vi "RSNRPZ Get Usage Map.vi"(8 "error in (no error)":errorcluster, 9 "Max Len (1024)":u32=1024) -> (0 "error out":errorcluster, 1 "Map":string, 2 "Ret Len":u32)   [LabVIEW 2010]
doc: "Starting with revision 3.2.1.0 of this driver, the underlying low level library has been made usable by multiple applications concurrently. A sensor which is already in use by another running application cannot by initialized by a different In this case the rsnrpz_init() function would return a status NRP_ERROR_SENSOR_IN_USE (0xC0000022). \n\nrsnrpz_getUsageMap() can be used to get a textual description of the current sensor & application relationship. For a sensor which is already in use, the application which holds the sensor, is shown in the usage map. This information can, for example, be presented to a user. \n\nThe textual usage map is returned via a char buffer 'Map' which should be supplied by the caller. 'maxLen' should be set to the size of the user's buffer in order to limit the amount of data which will be copied to 'map'.\nIf 'Ret Len' is not NULL, the current length of the usage map is returned here (which may be longer than 'Max Len'."
uses:
  rsnrpz_32.dll
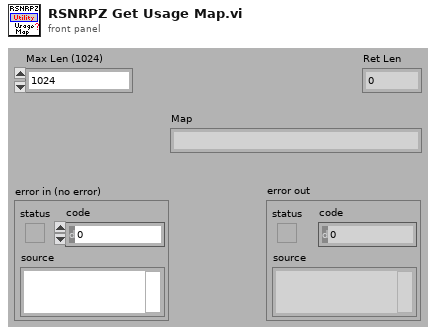
[diagram p1: front panel]
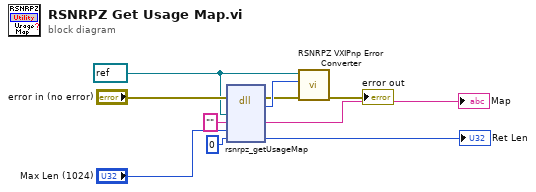
[diagram p0: block diagram]
diagram:
  w1 = refnum<visa-resource-name> refnum ("dup VISA session")
  n1 = dll-call lib="rsnrpz_32.dll" fn="rsnrpz_getUsageMap"(error in="error in (no error)", "Instrument Handle"=w1, "Map"="", "Max Len"="Max Len (1024)", "Ret Len"=u32 0) -> (error out=w4:errorcluster, w7:i32, "Map"=→"Map":string, "Ret Len"=→"Ret Len":u32)  [unwired: 4 in, 1 out]
  n2 = call <instrlib>:"RSNRPZ VXIPnp Error Converter.vi"("error in"=w4, "VXIPnp error code"=w7, "VISA session"=w1) -> ("error out"=→"error out":errorcluster)  [unwired: 7 in, 1 out]
